vi "direction_to_quaternion.vi"(8 "To":dbl[](array[numeric]), 11 "From":dbl[](array[numeric])) -> (2 "Quaternion":dbl[](array[numeric]))   [LabVIEW 2013]
uses:
  <vilib>/Analysis/baseanly.llb/Real Dot Product.vi
  norm_vec.vi
  magnitude_dbl.vi
  <vilib>/Analysis/NI_AALBase.lvlib
panel:
  # "Create a quaternion from two direction vectors (need not be normalized). The rotation maps the \"from\" vector onto the \"to\" vector, defining the unspecified rotation component so that there is no component of rotation about the \"from\" axis.  This is useful for pointing in a direction when we don't care about rotation around the axis (or we want it to be zero.)"
  # "w"
  # "x1"
  # "x2"
  # "x3"
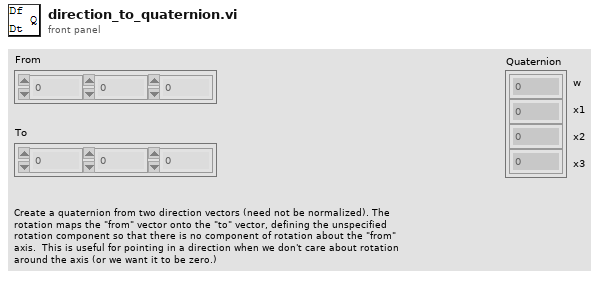
[diagram p1: front panel]
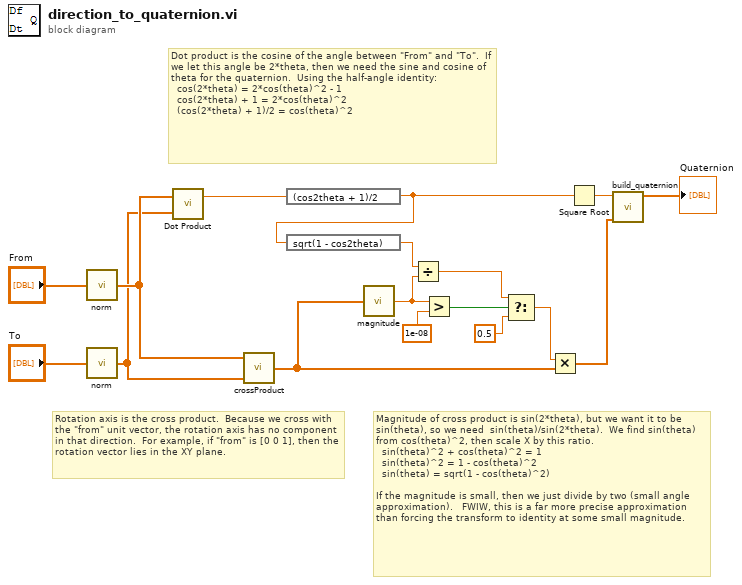
[diagram p0: block diagram]
diagram:
  # "Dot product is the cosine of the angle between \"From\" and \"To\".  If we let this angle be 2*theta, then we need the sine and cosine of theta for the quaternion.  Using the half-angle identity:\n  cos(2*theta) = 2*cos(theta)^2 - 1\n  cos(2*theta) + 1 = 2*cos(theta)^2 \n  (cos(2*theta) + 1)/2 = cos(theta)^2"
  # "Magnitude of cross product is sin(2*theta), but we want it to be sin(theta), so we need  sin(theta)/sin(2*theta).  We find sin(theta) from cos(theta)^2, then scale X by this ratio.  \n  sin(theta)^2 + cos(theta)^2 = 1\n  sin(theta)^2 = 1 - cos(theta)^2\n  sin(theta) = sqrt(1 - cos(theta)^2)\n\nIf the magnitude is small, then we just divide by two (small angle approximation).   FWIW, this is a far more precise approximation than forcing the transform to identity at some small magnitude."
  # "Rotation axis is the cross product.  Because we cross with the \"from\" unit vector, the rotation axis has no component in that direction.  For example, if \"from\" is [0 0 1], then the rotation vector lies in the XY plane."
  n1 = call-poly "norm.vi"("vector"="From") -> ("normalized vector"=w15:dbl[])  [unwired: 3 in, 1 out]
  n2 = call-poly "norm.vi"("vector"="To") -> ("normalized vector"=w14:dbl[])  [unwired: 3 in, 1 out]
  n3 = call-poly <vilib>:"Dot Product.vi"("Y Vector"=w14, "X Vector"=w15) -> ("X * Y"=w13:dbl)  [unwired: 1 out]
  n4 = call "crossProduct.vi"("B"=w14, "A"=w15) -> ("A x B"=w4:dbl[])  [unwired: 3 in]
  n5 = expression code="(cos2theta + 1)/2"(w13) -> (w11:dbl)
  n6 = expression code="sqrt(1 - cos2theta)"(w11) -> (w8:dbl)
  n7 = call-poly "magnitude.vi"("vector"=w4) -> ("vector magnitude"=w7:dbl)  [unwired: 4 in]
  n8 = Divide(x=w8, y=w7) -> (x/y=w6:dbl)
  n9 = Greater?(x=w7, y=1e-08) -> (0:w9:bool)
  n10 = Select(t=w6, s=w9, f=0.5 ("t")) -> (s? t:f=w3:dbl)
  n11 = Multiply(x=w3, y=w4) -> (x*y=w2:dbl[])
  n12 = Square Root(x=w11) -> (sqrt(x)=w12:dbl)
  n13 = call "build_quaternion.vi"("x"=w2, "w"=w12) -> ("Quaternion"=→"Quaternion":dbl[])  [unwired: 9 in]
